vi "Evaluate Pane Scroll.vi"(8 "error in (no error)":errorcluster, 11 "VI Reference":refnum<vi>) -> (0 "error out":errorcluster, 3 "Pane Scrolled":bool)   [LabVIEW 2017, in "Front Panel Publisher.lvlib"]
doc: "This VI will keep track of origin movement, or scrolling of panes within a front panel of a VI. Pass in the VI reference of the front panel to this VI and what will be returned is a boolean stating if the origin of a pane has changed since the last time this function has been called."
uses:
  Front Panel Publisher.lvlib
  <vilib>/Utility/miscctls.llb/LVPointTypeDef.ctl
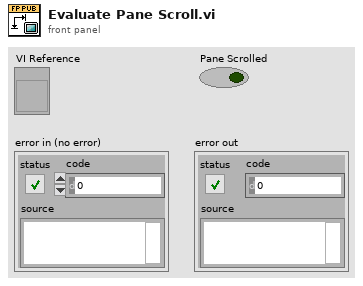
[diagram p1: front panel]
types:
  T1 = typedef "LVPointTypeDef.ctl" = cluster{"Horizontal":i16, "Vertical":i16}
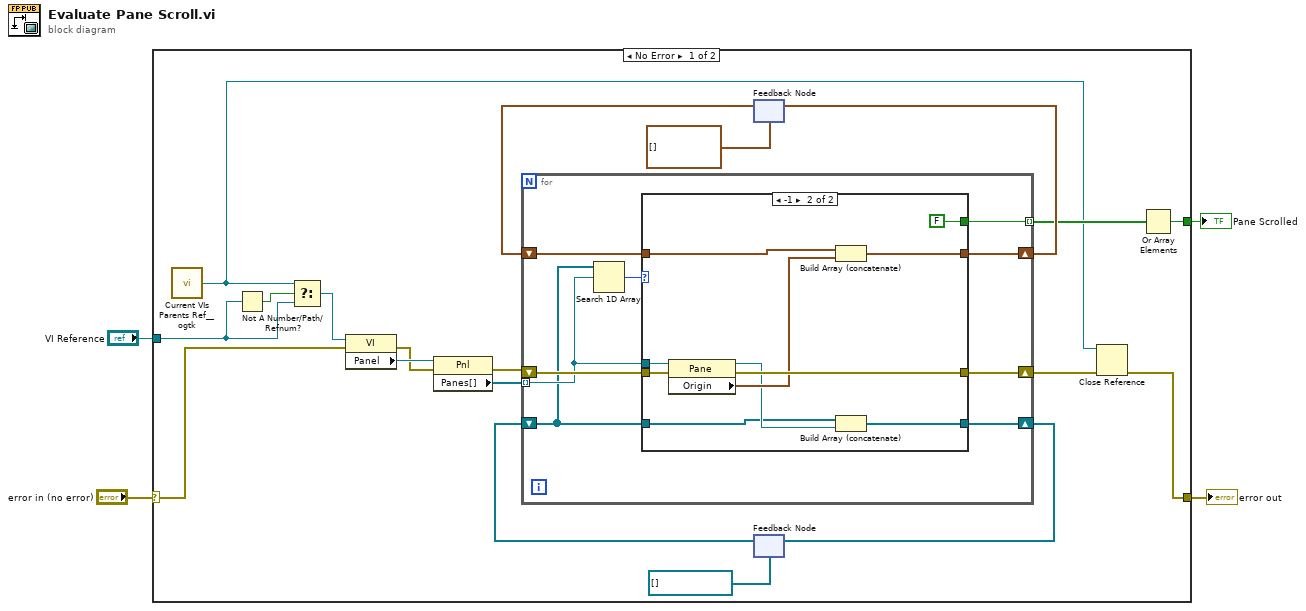
[diagram p0: block diagram]
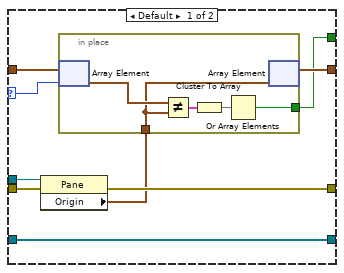
[diagram p2: hidden frame]
diagram:
  n1 = case shown="No Error" "error in (no error)" {
    selector: "error in (no error)" -> [w22 w57]
    tunnel: [w6 w57] -> w4
    tunnel: [w10 _] -> w2
    tunnel: "VI Reference" -> [w7 _]
    frame No Error {
      n2 = call <userlib>:"Current VIs Parents Ref__ogtk.vi"() -> ("Calling VI's Reference"=w5:refnum<vi>)  [unwired: 2 in]
      n3 = Not A Number/Path/Refnum?(number/path/refnum=w7) -> (NaN/Path/Refnum?=w9:bool)
      n4 = Select(t=w5, s=w9, f=w7) -> (s? t:f=w8:refnum<vi>)
      n5 = property class="VI"(reference=w8, error in=w22) -> (error out=w19:errorcluster, "Panel"=w20:refnum<vi>)  [unwired: 1 out]
      n6 = property class="Pnl"(reference=w20, error in=w19) -> (error out=w18:errorcluster, "Panes[]"=w21:refnum<vi>[])  [unwired: 1 out]
      n7 = feedback #1(T1[] []) -> (w16:T1[])
      n8 = feedback #2(refnum<vi>[] []) -> (w13:refnum<vi>[])
      n9 = for {
        tunnel: w21 -> [w30] mode=indexing
        shift-right: [w31] -> w23
        shift-left: w18 -> [w32]
        shift-right: [w28] -> w17
        shift-left: w16 -> [w27]
        tunnel: [w26] -> w11 mode=indexing
        shift-right: [w25] -> w14
        shift-left: w13 -> [w24]
        n10 = Search 1D Array(1D array=w24, element=w30) -> (index of element=w29:i32)  [unwired: 1 in]
        n11 = case shown="-1" w29 {
          selector: w29 -> [w36 _]
          tunnel: w32 -> [w40 w56]
          tunnel: [w38 w55] -> w31
          tunnel: w30 -> [w41 w54]
          tunnel: [w34 w52] -> w28
          tunnel: w27 -> [w37 w51]
          tunnel: [w33 FALSE] -> w26
          tunnel: [w39 w48] -> w25
          tunnel: w24 -> [w39 w47]
          frame Default {
            n12 = property class="Pane"(reference=w41, error in=w40) -> (error out=w38:errorcluster, "Origin"=w35:T1)  [unwired: 1 out]
            n13 = in-place {
              in-place-border: w35 -> [w43]
              in-place-border: [w42] -> w33
              n14 = in-place-array #3(w37, w36) -> (w44:T1)
              n15 = Not Equal?(x=w44, y=w43) -> (x != y?=w45:cluster{"Horizontal":bool, "Vertical":bool})
              n16 = Cluster To Array(cluster=w45) -> (array=w46:bool[])
              n17 = Or Array Elements(Boolean array=w46) -> (logical OR=w42:bool)
              n18 = in-place-array #3(w43) -> (w34:T1[])  [unwired: 1 out]
            }
          }
          frame -1 {
            n19 = property class="Pane"(reference=w54, error in=w56) -> (reference out=w49:refnum<vi>, error out=w55:errorcluster, "Origin"=w53:T1)
            n20 = Build Array (concatenate)(w51, w53) -> (w52:T1[])
            n21 = Build Array (concatenate)(w47, w49) -> (w48:refnum<vi>[])
          }
        }
      }
      n22 = feedback-in #1(w17) -> ()
      n23 = feedback-in #2(w14) -> ()
      n24 = Close Reference(reference=w5, error in (no error)=w23) -> (error out=w6:errorcluster)
      n25 = Or Array Elements(Boolean array=w11) -> (logical OR=w10:bool)
    }
    frame Error {
    }
  }
  "error out" <- w4
  "Pane Scrolled" <- w2
